vi "Format_Save(SubVI).vi"(6 "4 Col":string, 7 "1 Col":string, 8 "error in (no error)":errorcluster, 9 "3 Col":string, 10 "2 Col":string, 11 "refnum in":refnum<file>) -> (0 "error out":errorcluster, 3 "refnum out":refnum<file>)   [LabVIEW 2014]
doc: "This SubVI saving data to outter file in same format"
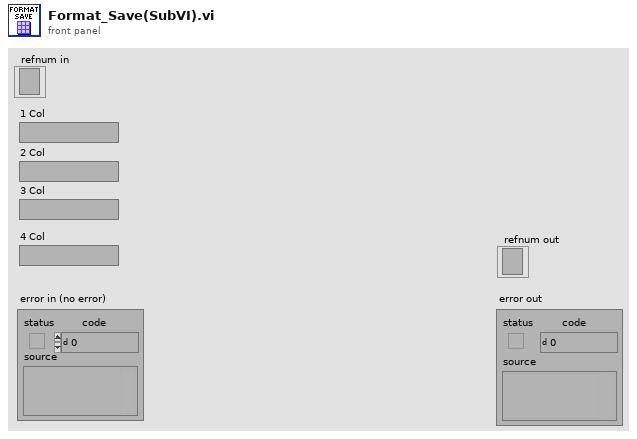
[diagram p1: front panel]
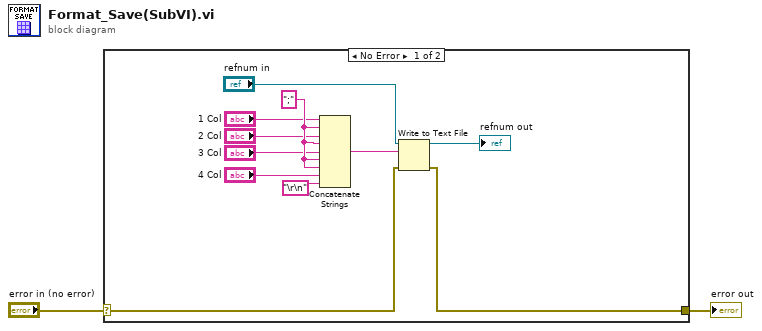
[diagram p0: block diagram]
diagram:
  n1 = case shown="No Error" "error in (no error)" {
    selector: "error in (no error)" -> [w10 w14]
    tunnel: [w9 w14] -> w1
    frame No Error {
      w13 = ";"
      n2 = Concatenate Strings("1 Col", w13, "2 Col", w13, "3 Col", w13, w13, "4 Col", "\r\n") -> (w12:string)
      n3 = Write to Text File(file (use dialog)="refnum in", text=w12, error in=w10) -> (refnum out=→"refnum out":refnum<file>, error out=w9:errorcluster)  [unwired: 1 in, 1 out]
    }
    frame Error {
    }
  }
  "error out" <- w1
